vi "change_status.vi"(8 "error in (no error)":errorcluster, 10 "String":string, 11 "String in":refnum<vi>) -> (0 "error out":errorcluster)   [LabVIEW 2017]
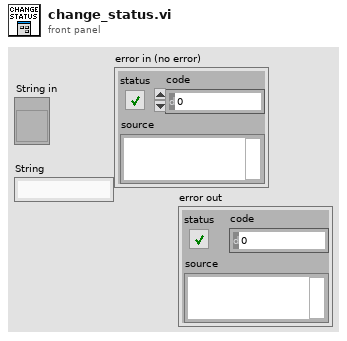
[diagram p1: front panel]
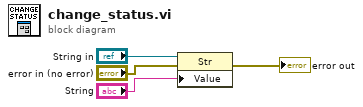
[diagram p0: block diagram]
diagram:
  n1 = property class="Str"(reference="String in", error in="error in (no error)", "Value"="String") -> (error out=→"error out":errorcluster)  [unwired: 1 out]
